vi "p1.vi"() -> ()   [LabVIEW 2021, in "d24.lvlib"]
uses:
  d24.lvlib
  7f23e7db-1a7a-4b44-a268-6fa00fde1ae0.vi
  AOC/AOC.lvlib
panel:
  out "XY Graph":cluster{i32[], i32[]}[](graph)=[{array[383928 elements], array[383928 elements]}, {[1, 4], [2, 4]}]
  in  "Example":string="#.######\n#>>.<^<#\n#.<..<<#\n#>v.><>#\n#<^v^^>#\n######.#"
  in  "Example":bool=TRUE
  out "Answer":i64=10
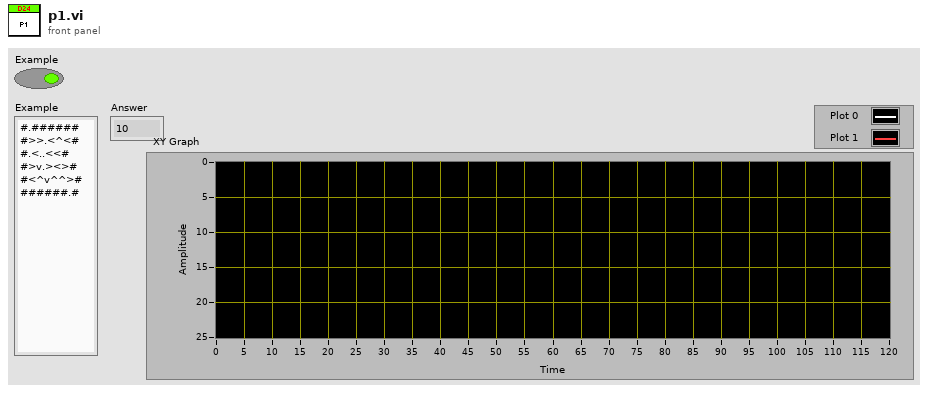
[diagram p1: front panel]
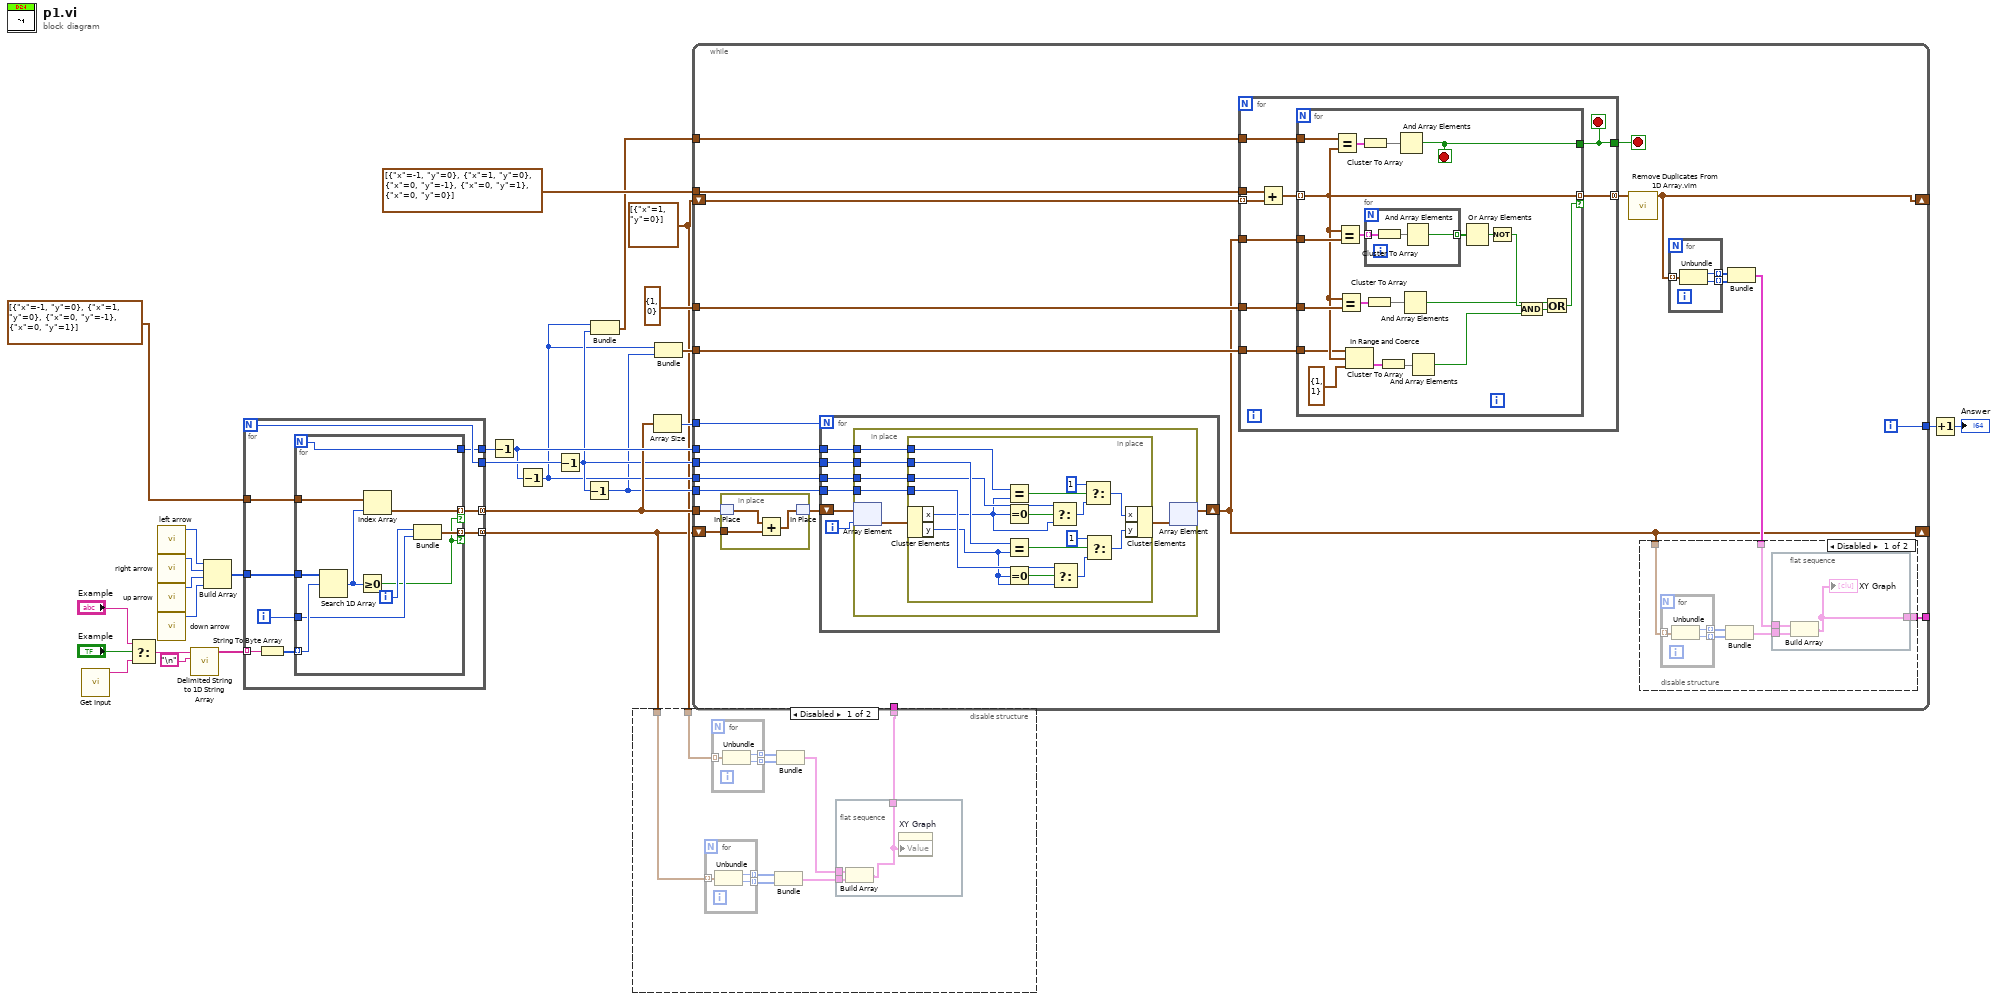
[diagram p0: block diagram]
diagram:
  w2 = cluster{"x":i32, "y":i32}[] [{"x"=1, "y"=0}]
  n1 = call "Get Input.vi"() -> ("Input"=w29:string)  [unwired: 11 in]
  n2 = Select(t="Example", s="Example", f=w29) -> (s? t:f=w28:string)
  n3 = call "left arrow.vi"() -> ("<"=w23:u8)  [unwired: 11 in]
  n4 = call "right arrow.vi"() -> (">"=w22:u8)  [unwired: 11 in]
  n5 = call "up arrow.vi"() -> ("^"=w21:u8)  [unwired: 11 in]
  n6 = call "down arrow.vi"() -> ("v"=w20:u8)  [unwired: 11 in]
  n7 = call <vilib>:"Delimited String to 1D String Array.vi"("delimiter"="\n", "delimited string"=w28) -> ("string array"=w24:string[])  [unwired: 9 in]
  n8 = Build Array(w23, w22, w21, w20) -> (w19:u8[])
  n9 = for {
    N -> [w34]
    tunnel: w24 -> [w38] mode=indexing
    tunnel: w19 -> [w36]
    tunnel: [w34] -> w17
    tunnel: [w33] -> w16
    tunnel: cluster{"x":i32, "y":i32}[] [{"x"=-1, "y"=0}, {"x"=1, "y"=0}, {"x"=0, "y"=-1}, {"x"=0, "y"=1}] -> [w32]
    tunnel: [w31] -> w10 mode=concatenating
    tunnel: [w30] -> w1 mode=concatenating
    i -> [w35]
    n10 = String To Byte Array(string=w38) -> (unsigned byte array=w37:u8[])
    n11 = for {
      N -> [w46]
      tunnel: w37 -> [w47] mode=indexing
      tunnel: w36 -> [w48]
      tunnel: w35 -> [w41]
      tunnel: [w46] -> w33
      tunnel: w32 -> [w45]
      tunnel: [w43] -> w31 mode=indexing if=w39
      tunnel: [w40] -> w30 mode=indexing if=w39
      i -> [w42]
      n12 = Search 1D Array(1D array=w48, element=w47) -> (index of element=w44:i32)  [unwired: 1 in]
      n13 = Greater Or Equal To 0?(x=w44) -> (x >= 0?=w39:bool)
      n14 = Index Array(array=w45, index=w44) -> (element=w43:cluster{"x":i32, "y":i32})
      n15 = Bundle(w42, w41) -> (w40:cluster{i32, i32})  [unwired: 1 in]
    }
  }
  n16 = Decrement(x=w16) -> (x-1=w15:i32)
  n17 = Decrement(x=w15) -> (x-1=w5:i32)
  n18 = Decrement(x=w17) -> (x-1=w8:i32)
  n19 = Decrement(x=w8) -> (x-1=w4:i32)
  n20 = Bundle(w5, w8) -> (w7:cluster{i32, i32})  [unwired: 1 in]
  n21 = disable-structure shown="Disabled" {
    disable-tunnel: [w55 _] -> w12
    disable-tunnel: w2 -> [w54 _]
    disable-tunnel: w1 -> [w49 _]
    frame Disabled {
      n22 = for {
        tunnel: w49 -> [w60] mode=indexing
        tunnel: [w59] -> w51 mode=indexing
        tunnel: [w58] -> w50 mode=indexing
        n23 = Unbundle(w60) -> (w59:i32, w58:i32)
      }
      n24 = for {
        tunnel: w54 -> [w63] mode=indexing
        tunnel: [w62] -> w53 mode=indexing
        tunnel: [w61] -> w52 mode=indexing
        n25 = Unbundle(w63) -> ("x"=w62:i32, "y"=w61:i32)
      }
      n26 = Bundle(w51, w50) -> (w57:cluster{i32[], i32[]})  [unwired: 1 in]
      n27 = Bundle(w53, w52) -> (w56:cluster{i32[], i32[]})  [unwired: 1 in]
      n28 = flat-sequence {
        tunnel: w57 -> [w64]
        tunnel: w56 -> [w66]
        tunnel: [w65] -> w55
        frame #0 {
          n29 = Build Array(w66, w64) -> (w65:cluster{i32[], i32[]}[])
          n30 = property on="XY Graph" class="XYGraph (strict)"("Value"=w65) -> ()  [unwired: 2 in, 2 out]
        }
      }
    }
    frame Enabled {
    }
  }
  n31 = Array Size(array=w10) -> (size(s)=w18:i32)
  n32 = Bundle(w5, w4) -> (w3:cluster{i32, i32})  [unwired: 1 in]
  n33 = while {
    tunnel: w18 -> [w88]
    tunnel: w8 -> [w86]
    tunnel: w15 -> [w87]
    tunnel: w5 -> [w85]
    tunnel: w4 -> [w84]
    tunnel: [w82] -> w14
    tunnel: [w80] -> _
    tunnel: w12 -> [_]
    tunnel: w10 -> [w78]
    shift-right: [w67] -> _
    shift-left: w1 -> [w77]
    shift-right: [w70] -> _
    shift-left: w2 -> [w76]
    tunnel: cluster{"x":i32, "y":i32}[] [{"x"=-1, "y"=0}, {"x"=1, "y"=0}, {"x"=0, "y"=-1}, {"x"=0, "y"=1}, {"x"=0, "y"=0}] -> [w75]
    tunnel: w7 -> [w74]
    tunnel: cluster{"x":i32, "y":i32} {"x"=1, "y"=0} ("Cluster") -> [w73]
    tunnel: w3 -> [w71]
    i -> [w82]
    stop <- w83 stop-if-true
    n34 = in-place {
      in-place-border: w77 -> [w104]
      n35 = in-place-match #1(w78) -> (w105:cluster{"x":i32, "y":i32}[])
      n36 = Add(x=w105, y=w104) -> (x+y=w106:cluster{i32, i32}[])
      n37 = in-place-match #1(w106) -> (w79:cluster{"x":i32, "y":i32}[])
    }
    n38 = for {
      N: w88 -> [_]
      tunnel: w86 -> [w113]
      tunnel: w87 -> [w112]
      tunnel: w85 -> [w111]
      tunnel: w84 -> [w110]
      shift-right: [w107] -> w67
      shift-left: w79 -> [w109]
      i -> [w108]
      n39 = in-place {
        in-place-border: w113 -> [w118]
        in-place-border: w112 -> [w119]
        in-place-border: w111 -> [w116]
        in-place-border: w110 -> [w117]
        n40 = in-place-array #2(w109, w108) -> (w115:cluster{"x":i32, "y":i32})
        n41 = in-place {
          in-place-border: w119 -> [w135]
          in-place-border: w118 -> [w134]
          in-place-border: w117 -> [w129]
          in-place-border: w116 -> [w124]
          n42 = in-place-cluster #3(w115) -> ("x"=w123:i32, "y"=w120:i32)
          n43 = Equal?(x=w135, y=w123) -> (x = y?=w125:bool)
          n44 = Equal To 0?(x=w123) -> (x = 0?=w126:bool)
          n45 = Equal?(x=w134, y=w120) -> (x = y?=w133:bool)
          n46 = Equal To 0?(x=w120) -> (x = 0?=w132:bool)
          n47 = Select(t=w124, s=w126, f=w123) -> (s? t:f=w128:i32)
          n48 = Select(t=w129, s=w132, f=w120) -> (s? t:f=w131:i32)
          n49 = Select(t=1, s=w125, f=w128) -> (s? t:f=w122:i32)
          n50 = Select(t=1, s=w133, f=w131) -> (s? t:f=w121:i32)
          n51 = in-place-cluster #3("x"=w122, "y"=w121) -> (w114:cluster{"x":i32, "y":i32})
        }
        n52 = in-place-array #2(w114) -> (w107:cluster{"x":i32, "y":i32}[])  [unwired: 1 out]
      }
    }
    n53 = for {
      tunnel: [w137] -> w83
      tunnel: w67 -> [w142]
      tunnel: w76 -> [w143] mode=indexing
      tunnel: w75 -> [w144]
      tunnel: w74 -> [w138]
      tunnel: w73 -> [w140]
      tunnel: [w141] -> w72 mode=concatenating
      tunnel: w71 -> [w136]
      stop <- w137 stop-if-true
      n54 = Add(x=w144, y=w143) -> (x+y=w139:cluster{"x":i32, "y":i32}[])
      n55 = for {
        tunnel: w139 -> [w150] mode=indexing
        tunnel: w142 -> [w162]
        tunnel: [w150] -> w141 mode=indexing if=w159
        tunnel: w140 -> [w156]
        tunnel: w138 -> [w152]
        tunnel: [w151] -> w137
        tunnel: w136 -> [w148]
        stop <- w151 stop-if-true
        n56 = Equal?(x=w152, y=w150) -> (x = y?=w153:cluster{bool, bool})
        n57 = Equal?(x=w150, y=w162) -> (x = y?=w163:cluster{"x":bool, "y":bool}[])
        n58 = Equal?(x=w150, y=w156) -> (x = y?=w155:cluster{"x":bool, "y":bool})
        n59 = In Range and Coerce(upper limit=w148, x=w150, lower limit=cluster{"x":i32, "y":i32} {"x"=1, "y"=1}) -> (In Range?=w147:cluster{"x":bool, "y":bool})  [unwired: 1 out]
        n60 = Cluster To Array(cluster=w153) -> (array=w154:bool[])
        n61 = for {
          tunnel: w163 -> [w168] mode=indexing
          tunnel: [w166] -> w164 mode=indexing
          n62 = Cluster To Array(cluster=w168) -> (array=w167:bool[])
          n63 = And Array Elements(Boolean array=w167) -> (logical AND=w166:bool)
        }
        n64 = Cluster To Array(cluster=w155) -> (array=w158:bool[])
        n65 = Cluster To Array(cluster=w147) -> (array=w146:bool[])
        n66 = And Array Elements(Boolean array=w154) -> (logical AND=w151:bool)
        n67 = And Array Elements(Boolean array=w158) -> (logical AND=w157:bool)
        n68 = And Array Elements(Boolean array=w146) -> (logical AND=w145:bool)
        n69 = Or Array Elements(Boolean array=w164) -> (logical OR=w161:bool)
        n70 = Not(x=w161) -> (.not. x?=w160:bool)
        n71 = And(x=w160, y=w145) -> (x .and. y?=w165:bool)
        n72 = Or(x=w157, y=w165) -> (x .or. y?=w159:bool)
      }
    }
    n73 = call "Remove Duplicates From 1D Array.vim"("array"=w72) -> ("array with duplicates removed"=w70:cluster{"x":i32, "y":i32}[])  [unwired: 10 in]
    n74 = for {
      tunnel: w70 -> [w103] mode=indexing
      tunnel: [w102] -> w69 mode=indexing
      tunnel: [w101] -> w68 mode=indexing
      n75 = Unbundle(w103) -> ("x"=w102:i32, "y"=w101:i32)
    }
    n76 = Bundle(w69, w68) -> (w81:cluster{i32[], i32[]})  [unwired: 1 in]
    n77 = disable-structure shown="Disabled" {
      disable-tunnel: w81 -> [w93 _]
      disable-tunnel: [w92 _] -> w80
      disable-tunnel: w67 -> [w89 _]
      frame Disabled {
        n78 = for {
          tunnel: w89 -> [w97] mode=indexing
          tunnel: [w96] -> w91 mode=indexing
          tunnel: [w95] -> w90 mode=indexing
          n79 = Unbundle(w97) -> ("x"=w96:i32, "y"=w95:i32)
        }
        n80 = Bundle(w91, w90) -> (w94:cluster{i32[], i32[]})  [unwired: 1 in]
        n81 = flat-sequence {
          tunnel: w94 -> [w100]
          tunnel: w93 -> [w99]
          tunnel: [w98] -> w92
          frame #0 {
            n82 = Build Array(w99, w100) -> (w98:cluster{i32[], i32[]}[])
            "XY Graph" <- w98
          }
        }
      }
      frame Enabled {
      }
    }
  }
  n83 = Increment(x=w14) -> (x+1=→"Answer":i32)
